vi "Get Last Known State.vi"(10 "Debug Data in":refnum<class "Debug Data.lvclass">, 11 "Debug State Analyzer in":refnum<class "Debug State Analyzer.lvclass">) -> (2 "Lifecycle State":string, 3 "Debug State Analyzer out":refnum<class "Debug State Analyzer.lvclass">)   [LabVIEW 2020, in "Debug State Analyzer.lvclass"]
uses:
  Debug State Analyzer.lvclass
  Debug State Analyzer.lvclass/Debug State Analyzer.ctl
  Debug Data/Debug Data.lvclass
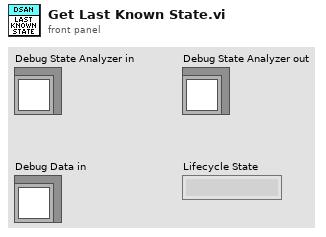
[diagram p1: front panel]
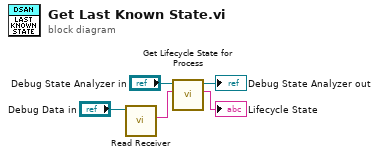
[diagram p0: block diagram]
diagram:
  n1 = call "Read Receiver.vi"("Debug Data In"="Debug Data in") -> ("Receiver"=w4:string)  [unwired: 9 in, 1 out]
  n2 = call "Get Lifecycle State for Process.vi"("Process"=w4, "Debug State Analyzer In"="Debug State Analyzer in") -> ("Lifecycle State"=→"Lifecycle State":string, "Debug State Analyzer Out"=→"Debug State Analyzer out":refnum<class "Debug State Analyzer.lvclass">)  [unwired: 8 in]
